vi "Channel Function.vi"   [LabVIEW 2017, in "Sefram DAS220.lvlib"]
doc: "A function can be applied on every channel to change unit (from voltage to bar for example) or to apply a mathematical predefined function."
uses:
  <instrlib>/Sefram DAS220/Sefram DAS220.lvlib
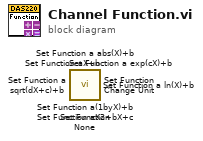
[diagram p0: block diagram]
diagram:
  n1 = call <instrlib>:"Set Function a(1byX)+b.vi"() -> ()  [unwired: 14 in, 2 out]
  n2 = call <instrlib>:"Set Function a exp(cX)+b.vi"() -> ()  [unwired: 14 in, 2 out]
  n3 = call <instrlib>:"Set Function a sqrt(dX+c)+b.vi"() -> ()  [unwired: 14 in, 2 out]
  n4 = call <instrlib>:"Set Function a ln(X)+b.vi"() -> ()  [unwired: 14 in, 2 out]
  n5 = call <instrlib>:"Set Function aX2+bX+c.vi"() -> ()  [unwired: 14 in, 2 out]
  n6 = call <instrlib>:"Set Function a abs(X)+b.vi"() -> ()  [unwired: 14 in, 2 out]
  n7 = call <instrlib>:"Set Function aX+b.vi"() -> ()  [unwired: 14 in, 2 out]
  n8 = call <instrlib>:"Set Function Change Unit.vi"() -> ()  [unwired: 14 in, 2 out]
  n9 = call <instrlib>:"Set Function None.vi"() -> ()  [unwired: 14 in, 2 out]
